vi "Parse 2D string values.vi"(11 "data string in":string) -> (1 "substring 2":string, 2 "image data":T1, 3 "new picture":picture)   [LabVIEW 2019]
uses:
  <vilib>/picture/picture.llb/imagedata.ctl
panel:
  out "Header":string
  out "data string out":string
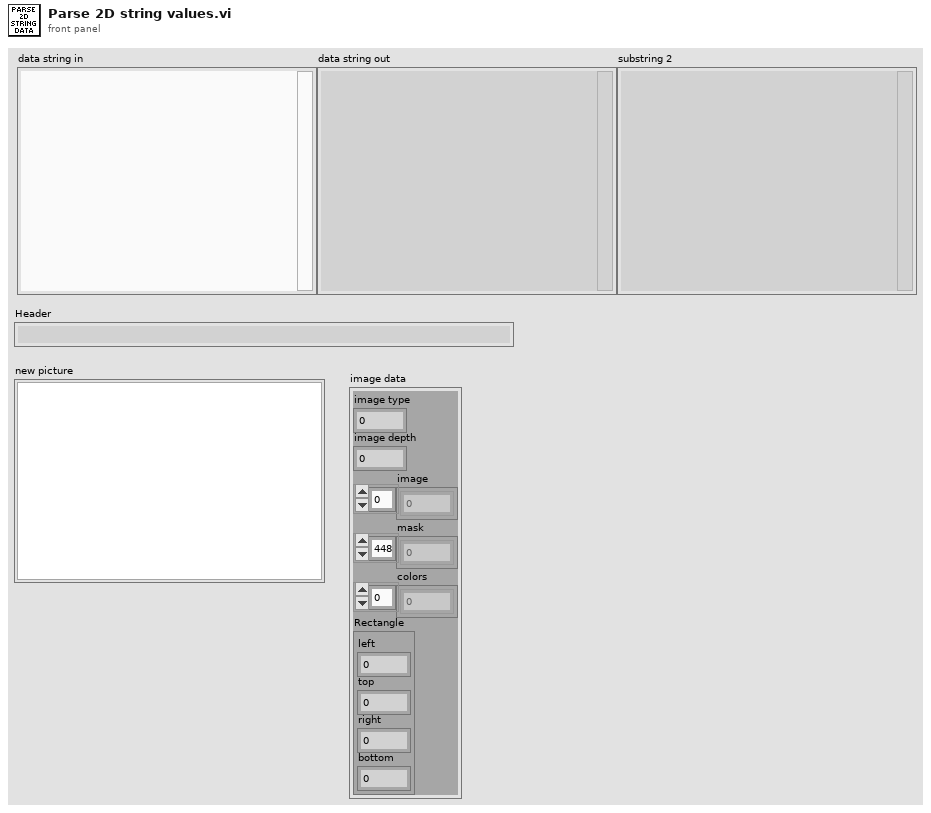
[diagram p1: front panel]
types:
  T1 = typedef "imagedata.ctl" = cluster{"image type":i32, "image depth":i32, "image":u8[], "mask":u8[], "colors":u32[], "Rectangle":cluster{"left":i16, "top":i16, "right":i16, "bottom":i16}}
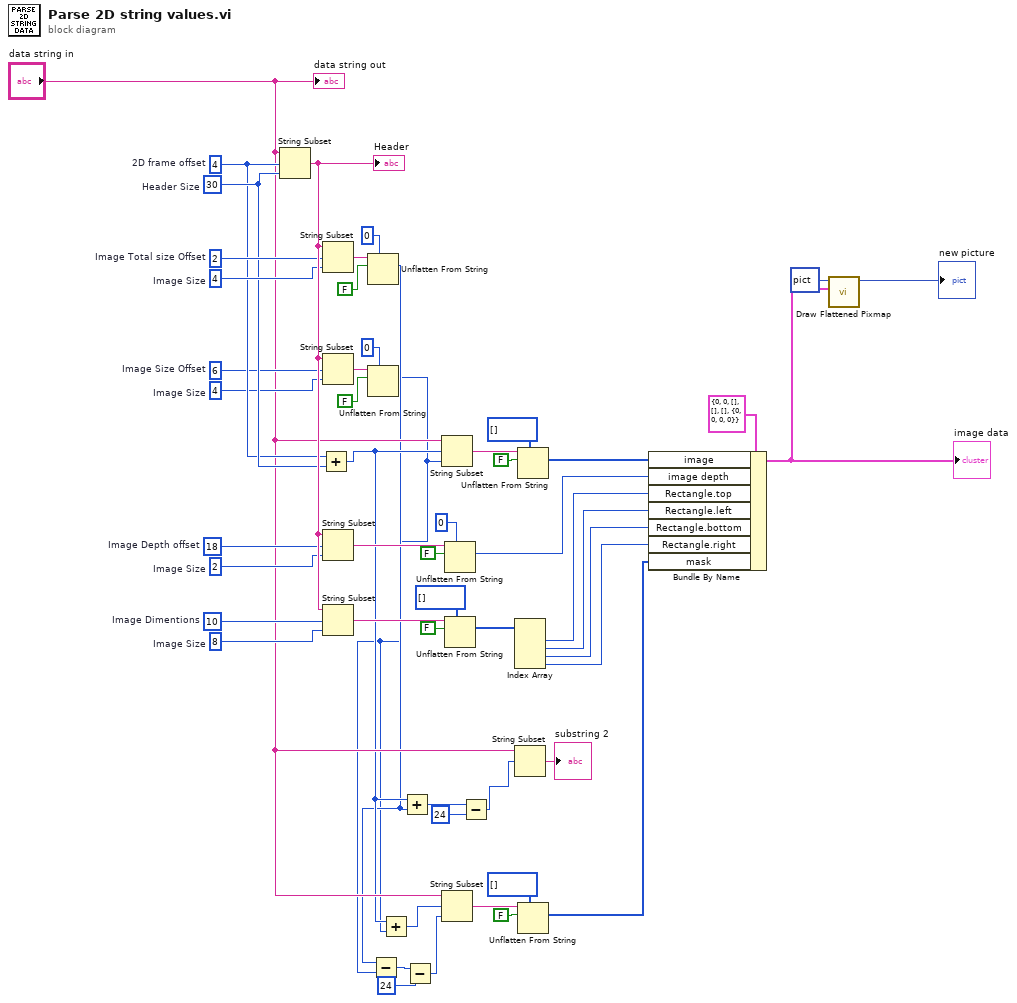
[diagram p0: block diagram]
diagram:
  w49 = 2  # Image Total size Offset
  w48 = 4  # Image Size
  w33 = 10  # Image Dimentions
  w34 = 8  # Image Size
  w25 = 18  # Image Depth offset
  w24 = 2  # Image Size
  w13 = 6  # Image Size Offset
  w14 = 4  # Image Size
  w17 = 4  # 2D frame offset
  w18 = 30  # Header Size
  n1 = String Subset(string="data string in", offset (0)=w17, length (rest)=w18) -> (substring=w50:string)
  "Header" <- w50
  n2 = Add(x=w17, y=w18) -> (x+y=w8:i32)
  n3 = String Subset(string=w50, offset (0)=w49, length (rest)=w48) -> (substring=w47:string)
  n4 = String Subset(string=w50, offset (0)=w13, length (rest)=w14) -> (substring=w15:string)
  n5 = String Subset(string=w50, offset (0)=w25, length (rest)=w24) -> (substring=w27:string)
  n6 = String Subset(string=w50, offset (0)=w33, length (rest)=w34) -> (substring=w32:string)
  n7 = Unflatten From String(type=0, binary string=w47, data includes array or string size? (T)=FALSE) -> (value=w5:i32)  [unwired: 2 in, 2 out]
  n8 = Unflatten From String(type=0, binary string=w15, data includes array or string size? (T)=FALSE) -> (value=w4:i32)  [unwired: 2 in, 2 out]
  n9 = Subtract(x=w5, y=w4) -> (x-y=w3:i32)
  n10 = Add(x=w8, y=w4) -> (x+y=w7:i32)
  n11 = Add(x=w8, y=w5) -> (x+y=w51:i32)
  n12 = Subtract(x=w3, y=24) -> (x-y=w2:i32)
  n13 = String Subset(string="data string in", offset (0)=w8, length (rest)=w4) -> (substring=w19:string)
  n14 = String Subset(string="data string in", offset (0)=w7, length (rest)=w2) -> (substring=w12:string)
  n15 = Unflatten From String(type=i16 0, binary string=w27, data includes array or string size? (T)=FALSE) -> (value=w30:i16)  [unwired: 2 in, 2 out]
  n16 = Unflatten From String(type=i16[] [], binary string=w32, data includes array or string size? (T)=FALSE) -> (value=w36:i16[])  [unwired: 2 in, 2 out]
  n17 = Subtract(x=w51, y=24) -> (x-y=w52:i32)
  n18 = Index Array(array=w36) -> (element #1=w37:i16, element #2=w38:i16, element #3=w39:i16, element #4=w40:i16)  [unwired: 4 in]
  n19 = String Subset(string="data string in", offset (0)=w52) -> (substring=→"substring 2":string)  [unwired: 1 in]
  n20 = Unflatten From String(type=u8[] [], binary string=w19, data includes array or string size? (T)=FALSE) -> (value=w23:u8[])  [unwired: 2 in, 2 out]
  n21 = Unflatten From String(type=u8[] [], binary string=w12, data includes array or string size? (T)=FALSE) -> (value=w6:u8[])  [unwired: 2 in, 2 out]
  n22 = Bundle By Name(cluster=T1 {"image type"=0, "image depth"=0, "image"=[], "mask"=[], "colors"=[], "Rectangle"={"left"=0, "top"=0, "right"=0, "bottom"=0}} ("image data"), "image"=w23, "image depth"=w30, "Rectangle.top"=w37, "Rectangle.left"=w38, "Rectangle.bottom"=w39, "Rectangle.right"=w40, "mask"=w6) -> (w43:T1)
  "image data" <- w43
  n23 = call <vilib>:"Draw Flattened Pixmap.vi"("image data"=w43, "picture"=picture data[5B]) -> ("new picture"=→"new picture":picture)  [unwired: 7 in]
  "data string out" <- "data string in"
